vi "Write header into the image.vi"(8 "error in (no error)":errorcluster, 11 "Save Image in":refnum<class "Save Image.lvclass">) -> (0 "error out":errorcluster, 3 "Save Image out":refnum<class "Save Image.lvclass">)   [LabVIEW 2018, in "Save Image.lvclass"]
uses:
  Save Image.lvclass
  Save Image.lvclass/Save Image.ctl
  Simulated_Header/Simulated_Header.lvclass/Simulated_Header.ctl
  Simulated_Header/Simulated_Header.lvclass
panel:
  out "Header Content":T1
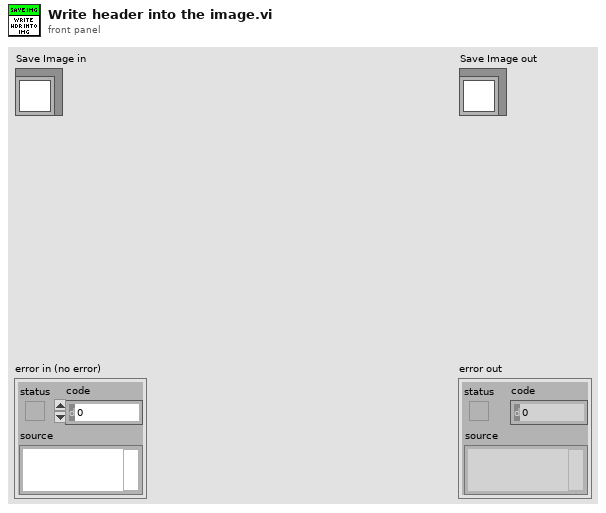
[diagram p1: front panel]
types:
  T1 = cluster{"FILENAME":cluster{"Name":string, "Value":string, "Comment":string}, "OBSERVER":cluster{"Name":string, "Value":string, "Comment":string}, "PROGRID":cluster{"Name":string, "Value":string, "Comment":string}, "OBJECT":cluster{"Name":string, "Value":string, "Comment":string}, "NIGHTDIR":cluster{"Name":string, "Value":string, "Comment":string}, "CHANNEL":cluster{"Name":string, "Value":string, "Comment":string}, "INSTRUME":cluster{"Name":string, "Value":string, "Comment":string}, "NEXPSEQ":cluster{"Name":string, "Value":string, "Comment":string}, "SEQINDEX":cluster{"Name":string, "Value":string, "Comment":string}, "OBSTYPE":cluster{"Name":string, "Value":string, "Comment":string}, "READMOD":cluster{"Name":string, "Value":string, "Comment":string}, "READMODE":cluster{"Name":string, "Value":string, "Comment":string}, "ACQMODE":cluster{"Name":string, "Value":string, "Comment":string}, "PREAMP":cluster{"Name":string, "Value":string, "Comment":string}, "READOUT":cluster{"Name":string, "Value":string, "Comment":string}, "VSHIFT":cluster{"Name":string, "Value":string, "Comment":string}, "TRIGGER":cluster{"Name":string, "Value":string, "Comment":string}, "EMMODE":cluster{"Name":string, "Value":string, "Comment":string}, "EMGAIN":cluster{"Name":string, "Value":string, "Comment":string}, "VBIN":cluster{"Name":string, "Value":string, "Comment":string}, "HBIN":cluster{"Name":string, "Value":string, "Comment":string}, "INITLIN":cluster{"Name":string, "Value":string, "Comment":string}, "INITCOL":cluster{"Name":string, "Value":string, "Comment":string}, "FINALLIN":cluster{"Name":string, "Value":string, "Comment":string}, "FINALCOL":cluster{"Name":string, "Value":string, "Comment":string}, "KSERLEN":cluster{"Name":string, "Value":string, "Comment":string}, "SHUTTER":cluster{"Name":string, "Value":string, "Comment":string}, "OPENSHT":cluster{"Name":string, "Value":string, "Comment":string}, "CLOSESHT":cluster{"Name":string, "Value":string, "Comment":string}, "DATE":cluster{"Name":string, "Value":string, "Comment":string}, "GAIN":cluster{"Name":string, "Value":string, "Comment":string}, "GAINERR":cluster{"Name":string, "Value":string, "Comment":string}, "RDNOISE":cluster{"Name":string, "Value":string, "Comment":string}, "RNOISERR":cluster{"Name":string, "Value":string, "Comment":string}, "SKYFIBER":cluster{"Name":string, "Value":string, "Comment":string}, "CALFIBER":cluster{"Name":string, "Value":string, "Comment":string}, "UTDATE":cluster{"Name":string, "Value":string, "Comment":string}, "LOCTIME":cluster{"Name":string, "Value":string, "Comment":string}, "MJD":cluster{"Name":string, "Value":string, "Comment":string}, "OBSLON":cluster{"Name":string, "Value":string, "Comment":string}, "OBSLAT":cluster{"Name":string, "Value":string, "Comment":string}, "OBSALT":cluster{"Name":string, "Value":string, "Comment":string}, "EXPTIME":cluster{"Name":string, "Value":string, "Comment":string}, "TELRA":cluster{"Name":string, "Value":string, "Comment":string}, "TELDEC":cluster{"Name":string, "Value":string, "Comment":string}, "RA":cluster{"Name":string, "Value":string, "Comment":string}, "DEC":cluster{"Name":string, "Value":string, "Comment":string}, "RA_DEG":cluster{"Name":string, "Value":string, "Comment":string}, "DEC_DEG":cluster{"Name":string, "Value":string, "Comment":string}, "EPOCH":cluster{"Name":string, "Value":string, "Comment":string}, "HA":cluster{"Name":string, "Value":string, "Comment":string}, "HAD":cluster{"Name":string, "Value":string, "Comment":string}, "AIRMASS":cluster{"Name":string, "Value":string, "Comment":string}, "AMSTART":cluster{"Name":string, "Value":string, "Comment":string}, "AMEND":cluster{"Name":string, "Value":string, "Comment":string}, "XOFFSET":cluster{"Name":string, "Value":string, "Comment":string}, "YOFFSET":cluster{"Name":string, "Value":string, "Comment":string}, "PA":cluster{"Name":string, "Value":string, "Comment":string}, "CAMFOC":cluster{"Name":string, "Value":string, "Comment":string}, "TELFOC":cluster{"Name":string, "Value":string, "Comment":string}, "TCSUT":cluster{"Name":string, "Value":string, "Comment":string}, "TCSST":cluster{"Name":string, "Value":string, "Comment":string}, "MOONDIST":cluster{"Name":string, "Value":string, "Comment":string}, "MOONALT":cluster{"Name":string, "Value":string, "Comment":string}, "MOONPHAS":cluster{"Name":string, "Value":string, "Comment":string}, "ADC":cluster{"Name":string, "Value":string, "Comment":string}, "ADCSPEED":cluster{"Name":string, "Value":string, "Comment":string}, "CALMIRR":cluster{"Name":string, "Value":string, "Comment":string}, "GUIDING":cluster{"Name":string, "Value":string, "Comment":string}, "GUIDTEXP":cluster{"Name":string, "Value":string, "Comment":string}, "GUIDFREQ":cluster{"Name":string, "Value":string, "Comment":string}, "GUIDOBJX":cluster{"Name":string, "Value":string, "Comment":string}, "GUIDOBJY":cluster{"Name":string, "Value":string, "Comment":string}, "AVGYCORR":cluster{"Name":string, "Value":string, "Comment":string}, "AVGXCORR":cluster{"Name":string, "Value":string, "Comment":string}, "GFOCUS":cluster{"Name":string, "Value":string, "Comment":string}, "THARLAMP":cluster{"Name":string, "Value":string, "Comment":string}, "HALLAMP":cluster{"Name":string, "Value":string, "Comment":string}, "AGITATOR":cluster{"Name":string, "Value":string, "Comment":string}, "THARMIRR":cluster{"Name":string, "Value":string, "Comment":string}, "DSTATUS":cluster{"Name":string, "Value":string, "Comment":string}, "DPOS":cluster{"Name":string, "Value":string, "Comment":string}, "DTEMP":cluster{"Name":string, "Value":string, "Comment":string}, "DHUM":cluster{"Name":string, "Value":string, "Comment":string}, "DLAMP":cluster{"Name":string, "Value":string, "Comment":string}, "DFLAT":cluster{"Name":string, "Value":string, "Comment":string}, "TEMPEXT":cluster{"Name":string, "Value":string, "Comment":string}, "PRESSURE":cluster{"Name":string, "Value":string, "Comment":string}, "HUMIDITY":cluster{"Name":string, "Value":string, "Comment":string}, "WINDDIR":cluster{"Name":string, "Value":string, "Comment":string}, "WINSPEED":cluster{"Name":string, "Value":string, "Comment":string}, "SHTTTL":cluster{"Name":string, "Value":string, "Comment":string}, "COOLER":cluster{"Name":string, "Value":string, "Comment":string}, "TEMP":cluster{"Name":string, "Value":string, "Comment":string}, "TEMPST":cluster{"Name":string, "Value":string, "Comment":string}, "SERN":cluster{"Name":string, "Value":string, "Comment":string}, "OBS_TITLE":cluster{"Name":string, "Value":string, "Comment":string}, "COMMENT":cluster{"Name":string, "Value":string, "Comment":string}, "SIMPLE":cluster{"Name":string, "Value":string, "Comment":string}, "NAXIS":cluster{"Name":string, "Value":string, "Comment":string}, "EXTEND":cluster{"Name":string, "Value":string, "Comment":string}}
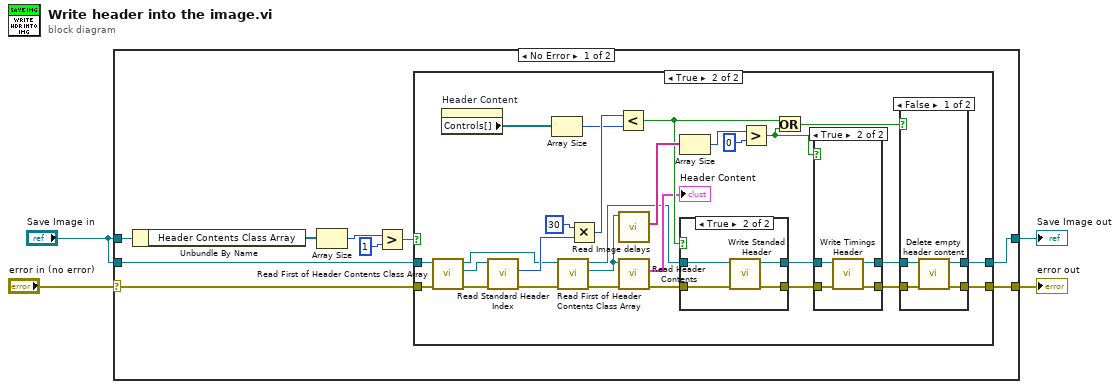
[diagram p0: block diagram]
diagram:
  n1 = case shown="No Error" "error in (no error)" {
    selector: "error in (no error)" -> [w6 w63]
    tunnel: [w13 w63] -> w3
    tunnel: [w12 w62] -> w2
    tunnel: "Save Image in" -> [w7 w62]
    tunnel: "Save Image in" -> [w5 _]
    frame No Error {
      n2 = Unbundle By Name(w7) -> ("Header Contents Class Array"=w11:refnum<class "Simulated_Header.lvclass">[])
      n3 = Array Size(array=w11) -> (size(s)=w10:i32)
      n4 = Greater?(x=w10, y=1) -> (0:w8:bool)
      n5 = case shown="True" w8 {
        tunnel: [w14 w43] -> w13
        tunnel: [w15 w42] -> w12
        tunnel: w6 -> [w14 w18]
        tunnel: w5 -> [w15 w22]
        frame False {
        }
        frame True {
          n6 = call "Read First of Header Contents Class Array.vi"("error in (no error)"=w18, "Save Image in"=w22) -> ("error out"=w17:errorcluster, "Simulated_Header.lvclass"=w16:refnum<class "Simulated_Header.lvclass">, "Save Image out"=w19:refnum<class "Save Image.lvclass">)  [unwired: 7 in]
          n7 = property on="Header Content" class="Clust (strict)"() -> ("Controls[]"=w26:refnum<vi>[])  [unwired: 2 in, 2 out]
          n8 = call "Read Standard Header Index.vi"("error in (no error)"=w17, "Simulated_Header in"=w16) -> ("error out"=w21:errorcluster, "Standard Header Index"=w20:u16)  [unwired: 7 in, 1 out]
          n9 = Array Size(array=w26) -> (size(s)=w39:i32)
          n10 = call "Read First of Header Contents Class Array.vi"("error in (no error)"=w21, "Save Image in"=w19) -> ("error out"=w25:errorcluster, "Simulated_Header.lvclass"=w24:refnum<class "Simulated_Header.lvclass">, "Save Image out"=w23:refnum<class "Save Image.lvclass">)  [unwired: 7 in]
          n11 = Multiply(x=30, y=w20) -> (x*y=w40:i32)
          n12 = Less?(x=w40, y=w39) -> (x < y?=w29:bool)
          n13 = call "Read Image delays.vi"("Header in"=w24) -> ("Image delays"=w37:string[])  [unwired: 8 in, 2 out]
          n14 = call "Read Header Contents.vi"("error in (no error)"=w25, "Header in"=w24) -> ("error out"=w38:errorcluster, "Header Content"=→"Header Content":T1)  [unwired: 7 in, 1 out]
          n15 = Array Size(array=w37) -> (size(s)=w36:i32)
          n16 = case shown="True" w29 {
            tunnel: w38 -> [w51 w54]
            tunnel: [w51 w52] -> w33
            tunnel: w23 -> [w50 w55]
            tunnel: [w50 w53] -> w34
            frame False {
            }
            frame True {
              n17 = call "Write Standad Header.vi"("error in (no error)"=w54, "Save Image in"=w55) -> ("error out"=w52:errorcluster, "Save Image out"=w53:refnum<class "Save Image.lvclass">)  [unwired: 8 in]
            }
          }
          n18 = Greater?(x=w36, y=0) -> (0:w30:bool)
          n19 = Or(x=w29, y=w30) -> (x .or. y?=w28:bool)
          n20 = case shown="True" w30 {
            tunnel: w33 -> [w45 w48]
            tunnel: [w45 w46] -> w31
            tunnel: w34 -> [w44 w49]
            tunnel: [w44 w47] -> w32
            frame False {
            }
            frame True {
              n21 = call "Write Timings Header.vi"("error in (no error)"=w48, "Save Image in"=w49) -> ("error out"=w46:errorcluster, "Save Image out"=w47:refnum<class "Save Image.lvclass">)  [unwired: 8 in]
            }
          }
          n22 = case shown="False" w28 {
            tunnel: w31 -> [w56 w61]
            tunnel: [w59 w61] -> w43
            tunnel: w32 -> [w57 w60]
            tunnel: [w58 w60] -> w42
            frame False {
              n23 = call "Delete empty header content.vi"("error in (no error)"=w56, "Save Image in"=w57) -> ("error out"=w59:errorcluster, "Save Image out"=w58:refnum<class "Save Image.lvclass">)  [unwired: 8 in]
            }
            frame True {
            }
          }
        }
      }
    }
    frame Error {
    }
  }
  "error out" <- w3
  "Save Image out" <- w2
